vi "Get CaseFrame Index By CaseName.vi"(8 "error in (no error)":errorcluster, 10 "CASE":string, 11 "CSM-Helper in":refnum<class "CSM-Helper.lvclass">) -> (0 "error out":errorcluster, 2 "index":i32, 3 "CSM-Helper out":refnum<class "CSM-Helper.lvclass">)   [LabVIEW 2020, in "CSM-Helper.lvclass"]
uses:
  CSM-Helper.lvclass
  CSM-Helper.lvclass/CSM-Helper.ctl
  Properties/Read Case Structure Ref.vi
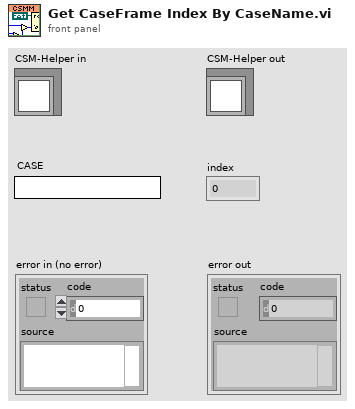
[diagram p1: front panel]
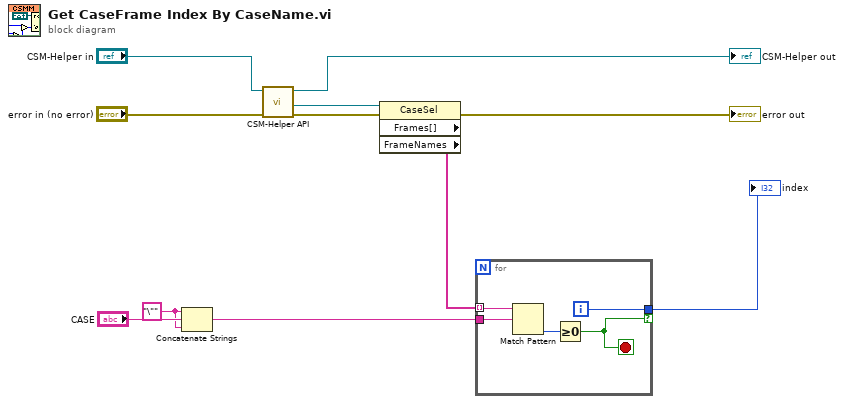
[diagram p0: block diagram]
diagram:
  w8 = "\"" ("string")
  n1 = Concatenate Strings(w8, "CASE", w8) -> (w9:string)
  n2 = call-poly "CSM-Helper API.vi"("error in (no error)"="error in (no error)", "CSM-Helper in"="CSM-Helper in") -> ("error out"=w2:errorcluster, "Case Structure"=w3:refnum<vi>, "CSM-Helper out"=→"CSM-Helper out":refnum<class "CSM-Helper.lvclass">)  [unwired: 7 in]
  n3 = property class="CaseSel" props=["Frames[]", "FrameNames"](reference=w3, error in=w2) -> (error out=→"error out":errorcluster, "FrameNames"=w11:string[])  [unwired: 2 out]
  n4 = for {
    tunnel: w11 -> [w16] mode=indexing
    tunnel: w9 -> [w15]
    tunnel: [w14] -> w4 if=w12
    i -> [w14]
    stop <- w12 stop-if-true
    n5 = Match Pattern(string=w16, regular expression=w15) -> (offset past match=w13:i32)  [unwired: 1 in, 3 out]
    n6 = Greater Or Equal To 0?(x=w13) -> (x >= 0?=w12:bool)
  }
  "index" <- w4
